vi "evenOdd.vi"(9 "String 2":string, 10 "A":dbl, 11 "String":string) -> (3 "String 3":string)   [LabVIEW 2021]
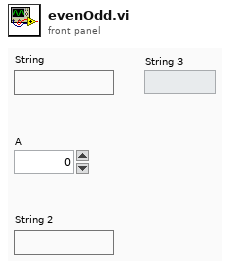
[diagram p1: front panel]
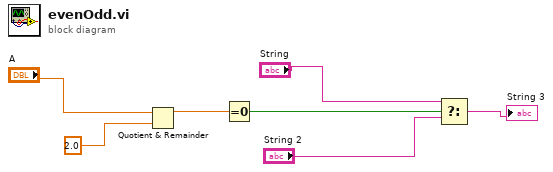
[diagram p0: block diagram]
diagram:
  n1 = Quotient & Remainder(x="A", y=2.0 ("floor(x/y)")) -> (x-y*floor(x/y)=w5:dbl)  [unwired: 1 out]
  n2 = Equal To 0?(x=w5) -> (x = 0?=w6:bool)
  n3 = Select(t="String", s=w6, f="String 2") -> (s? t:f=→"String 3":string)
